vi "Create Projection Plane.vi"(6 "Min":sgl, 7 "Plane":enum16{"X-Y Plane", "Y-Z Plane", "X-Z Plane"}(ring), 8 "error out (no error)":errorcluster, 9 "Origin Plot Ref":refnum<vi>) -> (0 "error out":errorcluster, 1 "Dup Origin Plot Ref":refnum<vi>, 3 "Projection Object Ref":refnum<vi>)   [LabVIEW 2017, in "3D Plot.lvclass"]
uses:
  <vilib>/Math Plots/3D Math Plots/3D Plot/3D Plot/3D Plot.lvclass
  <vilib>/picture/3D Picture Control/Object/Create Object (name).vi
  <vilib>/picture/3D Picture Control/NI_3D Picture Control.lvlib
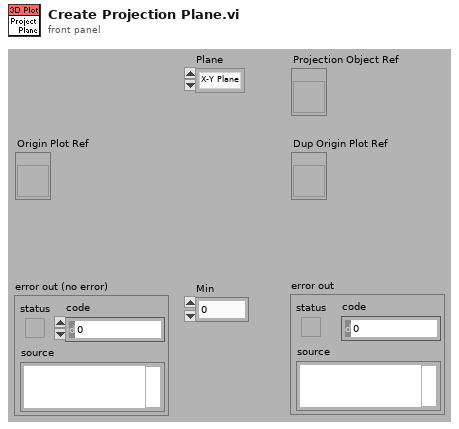
[diagram p1: front panel]
types:
  T1 = enum16{"Inherit Value", "Points", "Wireframe", "Polygons"}
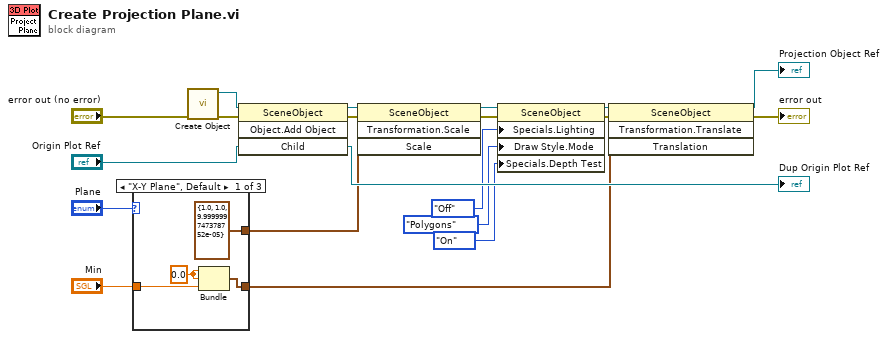
[diagram p0: block diagram]
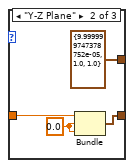
[diagram p2: hidden frame]
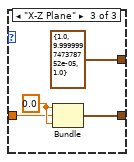
[diagram p3: hidden frame]
diagram:
  n1 = case shown="\"X-Y Plane\", Default" "Plane" {
    tunnel: [cluster{"X":sgl, "Y":sgl, "Z":sgl} {"X"=1.0, "Y"=1.0, "Z"=0.0001} ("Scale") cluster{"X":sgl, "Y":sgl, "Z":sgl} {"X"=0.0001, "Y"=1.0, "Z"=1.0} ("Scale") cluster{"X":sgl, "Y":sgl, "Z":sgl} {"X"=1.0, "Y"=0.0001, "Z"=1.0} ("Scale")] -> w2
    tunnel: "Min" -> [w22 w26 w29]
    tunnel: [w21 w25 w30] -> w1
    frame "X-Y Plane", Default {
      w23 = sgl 0.0 ("Minimum")
      n2 = Bundle("Minimum"=w23, "Minimum"=w23, "Min"=w22) -> (w21:cluster{"Minimum":sgl, "Minimum":sgl, "Min":sgl})  [unwired: 1 out]
    }
    frame "Y-Z Plane" {
      w27 = sgl 0.0 ("Minimum")
      n3 = Bundle("Min"=w26, "Minimum"=w27, "Minimum"=w27) -> (w25:cluster{"Min":sgl, "Minimum":sgl, "Minimum":sgl})  [unwired: 1 out]
    }
    frame "X-Z Plane" {
      w31 = sgl 0.0 ("Minimum")
      n4 = Bundle("Minimum"=w31, "Min"=w29, "Minimum"=w31) -> (w30:cluster{"Minimum":sgl, "Min":sgl, "Minimum":sgl})  [unwired: 1 out]
    }
  }
  n5 = call-poly <vilib>:"Create Object.vi"("error in (no error)"="error out (no error)") -> ("error out"=w10:errorcluster, "Scene:New Object"=w8:refnum<vi>)  [unwired: 9 in]
  n6 = invoke class="SceneObject" method="Object.Add Object"(reference=w8, error in=w10, "Child"="Origin Plot Ref") -> (reference out=w4:refnum<vi>, error out=w11:errorcluster, "Child"=→"Dup Origin Plot Ref":refnum<vi>)  [unwired: 1 in, 1 out]
  n7 = invoke class="SceneObject" method="Transformation.Scale"(reference=w4, error in=w11, "Scale"=w2) -> (reference out=w3:refnum<vi>, error out=w12:errorcluster)  [unwired: 1 in, 2 out]
  n8 = property class="SceneObject"(reference=w3, error in=w12, "Specials.Lighting"=enum16{"Inherit Value", "Off", "On"}."Off" ("Specials:Lighting"), "Draw Style.Mode"=T1."Polygons" ("Draw Style:Mode"), "Specials.Depth Test"=enum16{"Inherit Value", "Off", "On"}."On" ("Specials:Depth Test")) -> (reference out=w9:refnum<vi>, error out=w13:errorcluster)
  n9 = invoke class="SceneObject" method="Transformation.Translate"(reference=w9, error in=w13, "Translation"=w1) -> (reference out=→"Projection Object Ref":refnum<vi>, error out=→"error out":errorcluster)  [unwired: 1 in, 2 out]
